vi "-8342 Invalid Index--error.vi"(8 "error in":errorcluster, 11 "Index":string) -> (0 "error out":errorcluster)   [LabVIEW 2021, in "Open Xml.lvlib"]
uses:
  Open Xml.lvlib
  Common-LabVIEW-Helpers/Source/Error Helpers.lvlib
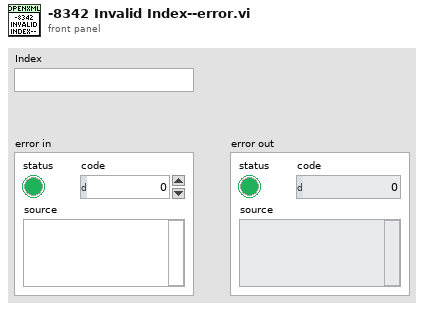
[diagram p1: front panel]
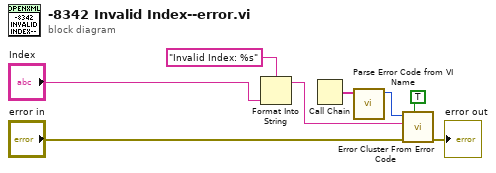
[diagram p0: block diagram]
diagram:
  n1 = Format Into String(format string="Invalid Index: %s" ("source"), "Index") -> (resulting string=w3:string)  [unwired: 2 in, 1 out]
  n2 = Call Chain() -> (call chain=w5:string[])
  n3 = call "Parse Error Code from VI Name.vi"("Call Chain"=w5) -> ("Error Code"=w4:i32)  [unwired: 10 in]
  n4 = call <vilib>:"Error Cluster From Error Code.vi"("show call chain? (False)"=TRUE, "error in (no error)"="error in", "error message (\"\")"=w3, "error code (0)"=w4) -> ("error out"=→"error out":errorcluster)  [unwired: 5 in]
